vi "Configure Active Reactive Current Limits.vi"(0 "VISA resource name":refnum<visa-resource-name>, 5 "Active Reactive Current Low Limit (0.0)":dbl min=0.0 max=6000.0 format="%.1f", 7 "Active Reactive Current High Limit (1000.0)":dbl=1000.0 min=0.0 max=1000.0 format="%.1f", 11 "error in (no error)":errorcluster) -> (4 "VISA resource name out":refnum<visa-resource-name>, 15 "error out":errorcluster)   [LabVIEW 2016, in "APT 300XAC Series.lvlib"]
doc: "Configures the <B>Frequency Limits</B> of the power source instrument used for testing.\n\n<B>Range</B> : 40.0~1000.0 Hz\n\nNote : Only supported in manual mode.\n\nThe Frequency Low-Limit defines the lower frequency limit of the output signal frequency APT300xAC Series Power Source can reach in Hz. Not reaching this value will fail the test\n\nThe Frequency High-Limit defines the higher frequency limit of the output signal frequency APT300xAC Series Power Source can reach in Hz. Crossing this value will fail the test"
uses:
  APT 300XAC Series.lvlib
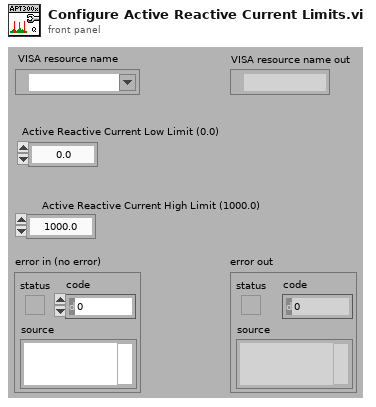
[diagram p1: front panel]
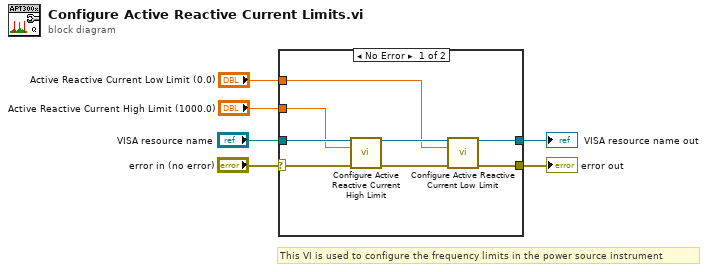
[diagram p0: block diagram]
diagram:
  # "This VI is used to configure the frequency limits in the power source instrument"
  n1 = case shown="No Error" "error in (no error)" {
    selector: "error in (no error)" -> [w12 w15]
    tunnel: "VISA resource name" -> [w14 w16]
    tunnel: [w8 w16] -> w5
    tunnel: [w7 w15] -> w4
    tunnel: "Active Reactive Current High Limit (1000.0)" -> [w13 _]
    tunnel: "Active Reactive Current Low Limit (0.0)" -> [w9 _]
    frame No Error {
      n2 = call "Configure Active Reactive Current High Limit.vi"("VISA resource name"=w14, "Active Reactive Current High Limit"=w13, "error in (no error)"=w12) -> ("VISA resource name out"=w11:refnum<visa-resource-name>, "error out"=w10:errorcluster)  [unwired: 11 in]
      n3 = call "Configure Active Reactive Current Low Limit.vi"("VISA resource name"=w11, "Active Reactive Current Low Limit"=w9, "error in (no error)"=w10) -> ("VISA resource name out"=w8:refnum<visa-resource-name>, "error out"=w7:errorcluster)  [unwired: 11 in]
    }
    frame Error {
    }
  }
  "error out" <- w4
  "VISA resource name out" <- w5
